vi "Mojo Engine.vi"(0 "Mojo Notifier":string, 11 "COM Port":string[](array[string])) -> ()   [LabVIEW 2020]
uses:
  FPGA Controls/FPGA Cluster.ctl
  FPGA Controls/FPGA Laser Mode.ctl
  FPGA Controls/FPGA Sequence Mode.ctl
  FPGA Controls/FPGA Notifier Element.ctl
  FPGA Controls/FPGA Action.ctl
panel:
  in  "488":T1 {"Duration digital" max=65535 step=1; "Duration slide" max=65535 step=1 scale=0.0..65535.0 scale format="%d us"; "Laser Mode" items=["Off", "On", "Rising", "Falling", "Camera"]}
  in  "405":T1 {"Duration digital" max=65535 step=1; "Duration slide" max=65535 step=1 scale=0.0..65535.0 scale format="%d us"; "Laser Mode" items=["Off", "On", "Rising", "Falling", "Camera"]}
  out "Startup Error":errorcluster
  in  "Quit":bool
  out "Version":u32
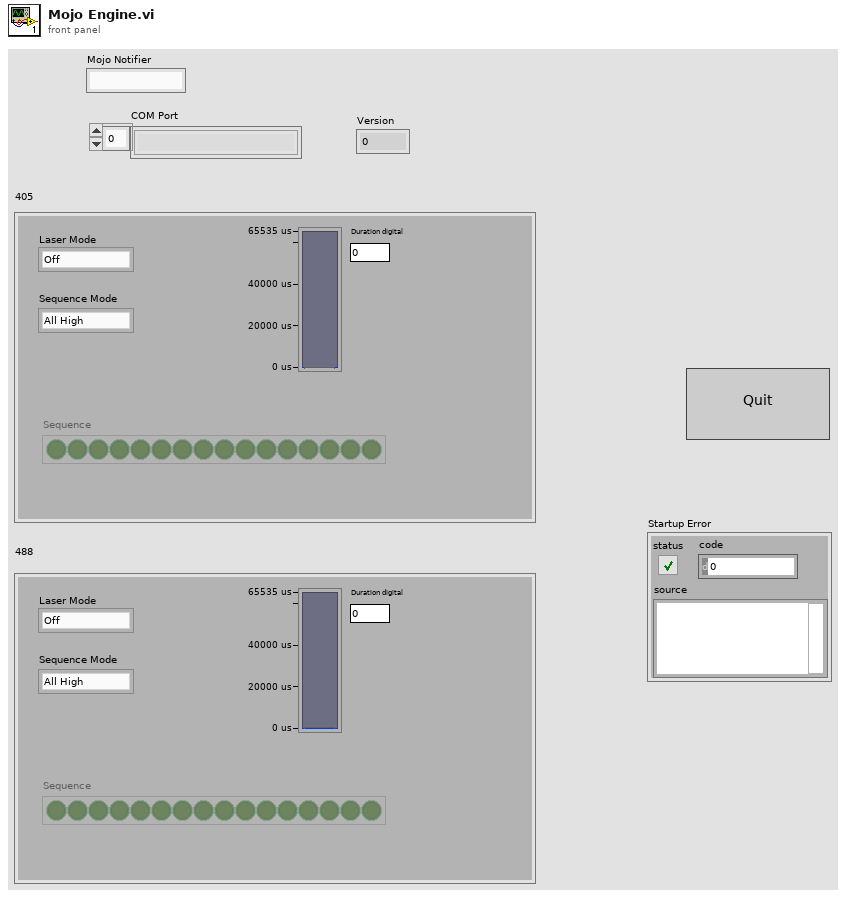
[diagram p1: front panel]
types:
  T1 = typedef "FPGA Cluster.ctl" = cluster{"Laser Mode":T2, "Sequence Mode":T3, "Duration slide":u32, "Duration digital":u32, "Sequence":bool[]}
  T2 = typedef "FPGA Laser Mode.ctl" = u16
  T3 = typedef "FPGA Sequence Mode.ctl" = enum16{"All High", "All Low", "Alternate 1010", "Alternate 0101", "Custom"}
  T4 = enum8{"Enabled", "Disabled", "Disabled and Grayed Out"}
  T5 = typedef "FPGA Notifier Element.ctl" = cluster{"Sequence":bool[], "Laser Mode":T2, "Duration":u32, "Laser Channel":u16, "Write Confirm ":bool, "Received?":bool, "FPGA Action":T6}
  T6 = typedef "FPGA Action.ctl" = enum16{"Set Laser Mode", "Set Sequence", "Set Duration", "Write Check", "Idle", "Quit"}
  T7 = enum16{"All High", "All Low", "Alternate 1010", "Alternate 0101", "Custom"}
  T8 = cluster{"Laser Mode":bool, "Sequence Mode":bool, "Duration slide":bool, "Duration digital":bool, "Sequence":bool[]}
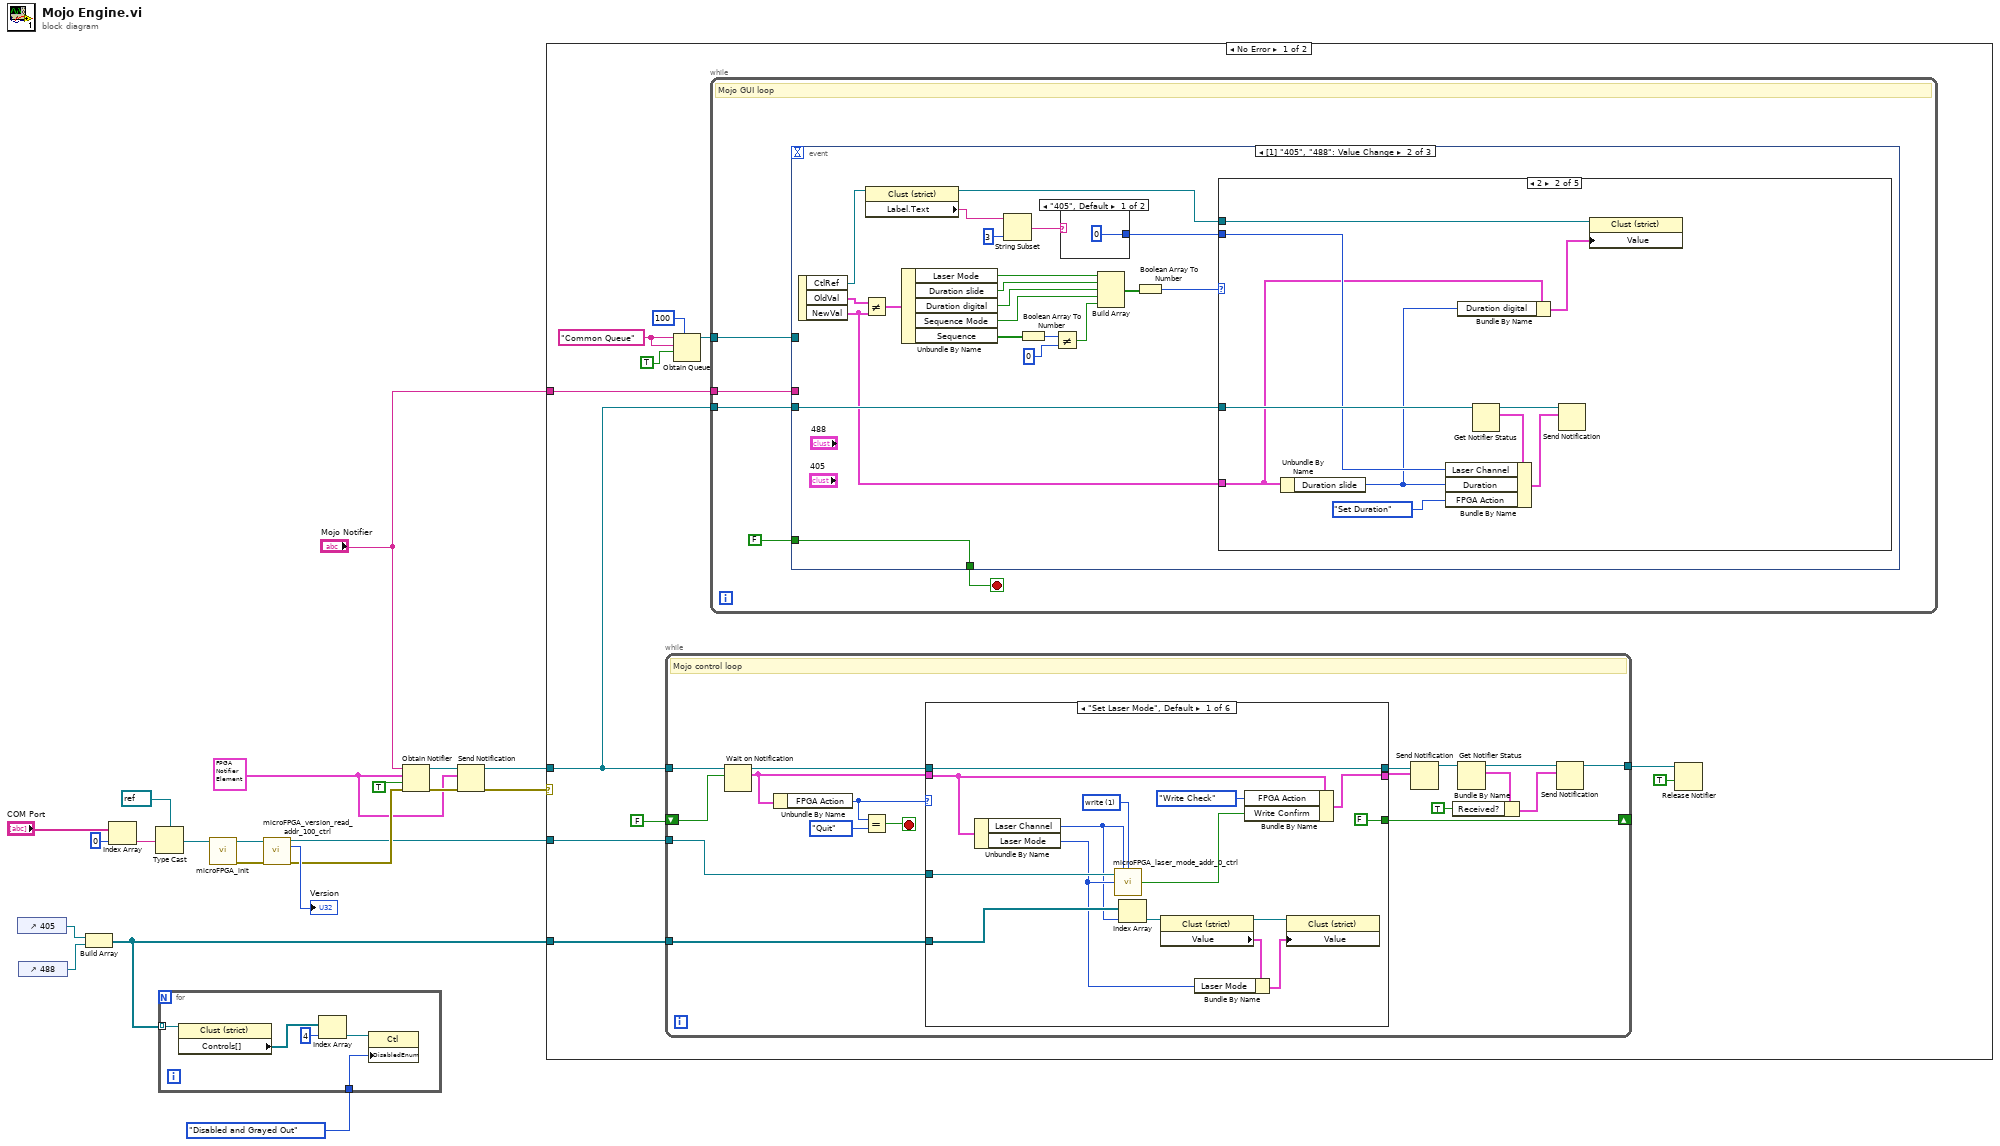
[diagram p0: block diagram]
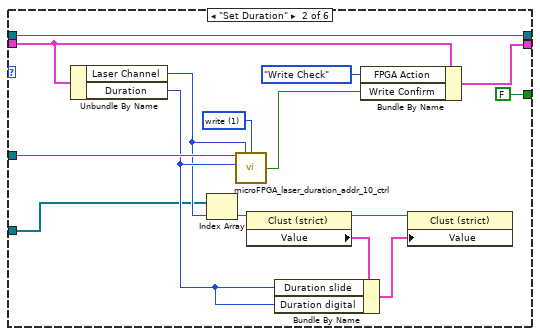
[diagram p2: hidden frame]
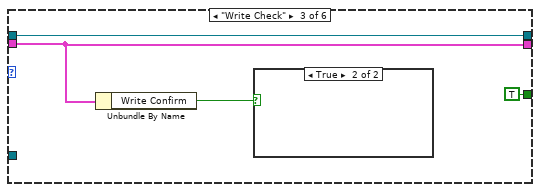
[diagram p3: hidden frame]
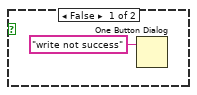
[diagram p4: hidden frame]
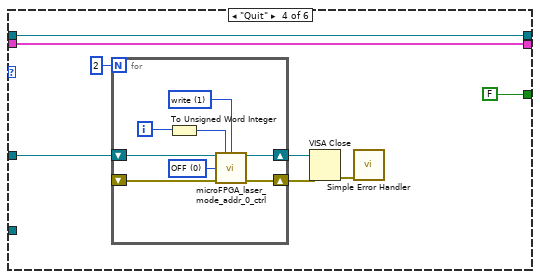
[diagram p5: hidden frame]
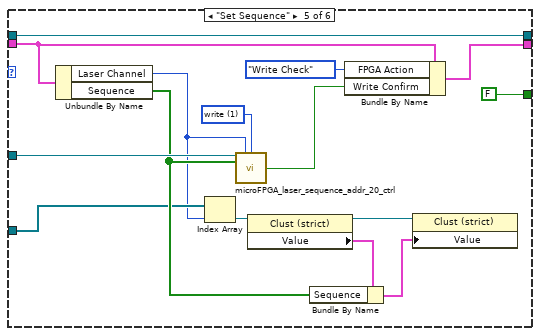
[diagram p6: hidden frame]
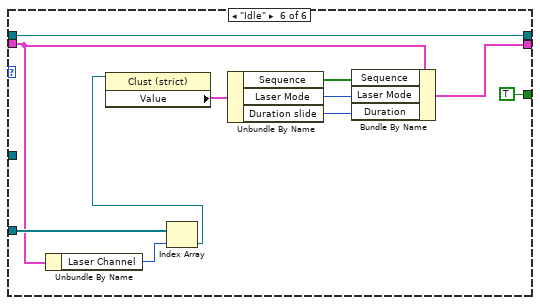
[diagram p7: hidden frame]
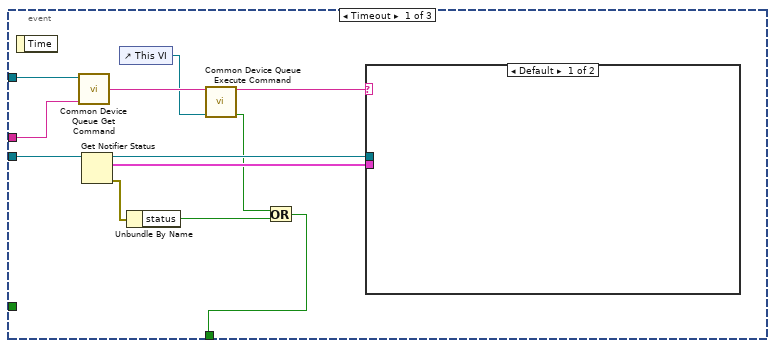
[diagram p8: hidden frame]
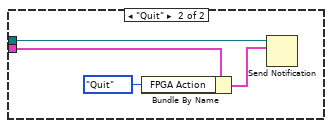
[diagram p9: hidden frame]
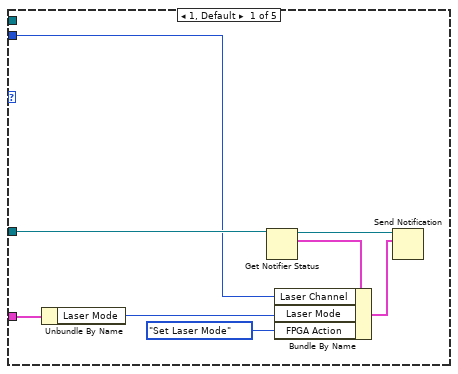
[diagram p10: hidden frame]
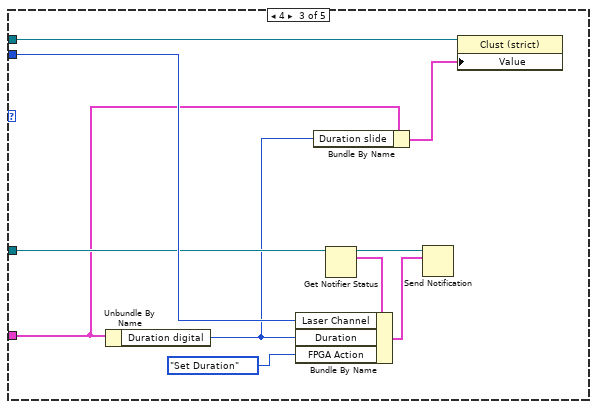
[diagram p11: hidden frame]
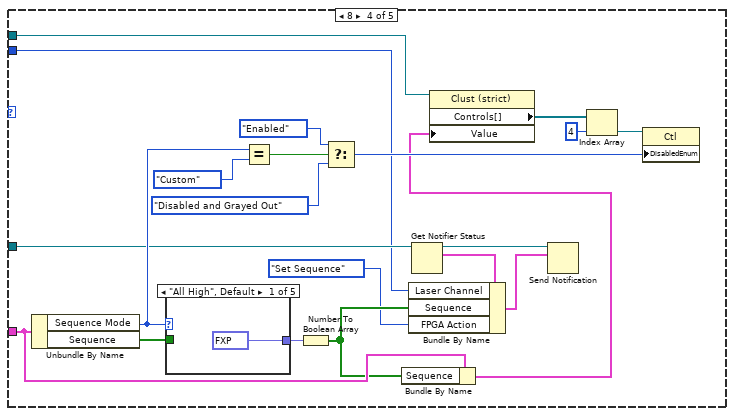
[diagram p12: hidden frame]
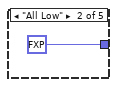
[diagram p13: hidden frame]
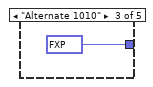
[diagram p14: hidden frame]
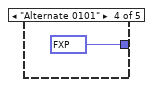
[diagram p15: hidden frame]
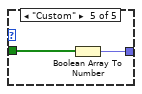
[diagram p16: hidden frame]
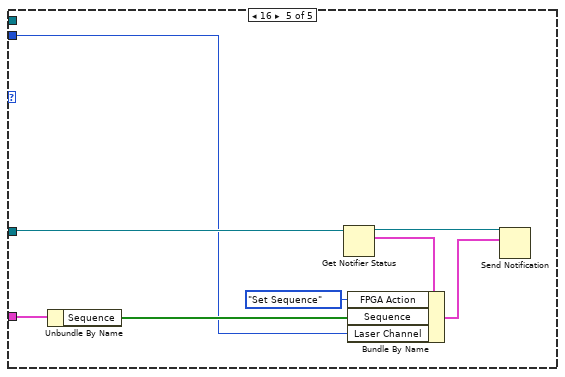
[diagram p17: hidden frame]
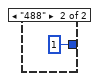
[diagram p18: hidden frame]
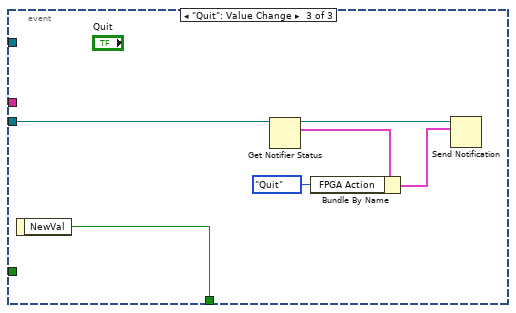
[diagram p19: hidden frame]
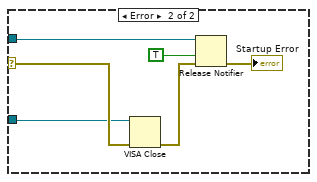
[diagram p20: hidden frame]
diagram:
  w5 = T5 {"Sequence"=[FALSE, FALSE, FALSE, FALSE, FALSE, FALSE, FALSE, FALSE, FALSE, FALSE, FALSE, FALSE, FALSE, FALSE, FALSE, FALSE], "Laser Mode"=0, "Duration"=0, "Laser Channel"=0, "Write Confirm "=FALSE, "Received?"=FALSE, "FPGA Action"=enum."Idle"} ("Mojo Notifier Element")
  n1 = control-ref of="405"() -> (w4:refnum<vi>)
  n2 = control-ref of="488"() -> (w3:refnum<vi>)
  n3 = Build Array(w4, w3) -> (w1:refnum<vi>[])
  n4 = Index Array(array="COM Port", index=0) -> (element=w19:string)
  n5 = Type Cast(type=refnum<visa-resource-name> refnum ("VISA resource name"), x=w19) -> (*(type *) &x=w17:refnum<visa-resource-name>)
  n6 = for {
    tunnel: w1 -> [w24] mode=indexing
    tunnel: T4."Disabled and Grayed Out" ("Disabled") -> [w22]
    n7 = property class="Clust (strict)"(reference=w24) -> ("Controls[]"=w23:refnum<vi>[])  [unwired: 1 in, 2 out]
    n8 = Index Array(array=w23, index=4) -> (element=w25:refnum<vi>)
    n9 = property class="Ctl"(reference=w25, "DisabledEnum"=w22) -> ()  [unwired: 1 in, 2 out]
  }
  n10 = call "microFPGA_init.vi"("VISA resource name"=w17) -> ("error out"=w15:errorcluster, "VISA resource name out"=w16:refnum<visa-resource-name>)  [unwired: 9 in]
  n11 = call "microFPGA_version_read_addr_100_ctrl.vi"("VISA resource name"=w16, "error in (no error)"=w15) -> ("VISA resource name out"=w7:refnum<visa-resource-name>, "Version"=→"Version":u32, "error out"=w13:errorcluster)  [unwired: 11 in]
  n12 = Obtain Notifier(name (unnamed)="Mojo Notifier", notification data type=w5, create if not found? (T)=TRUE, error in (no error)=w13) -> (notifier out=w11:refnum<notifier>, error out=w10:errorcluster)  [unwired: 1 out]
  n13 = Send Notification(notification=w5, notifier=w11, error in (no error)=w10) -> (notifier out=w8:refnum<notifier>, error out=w9:errorcluster)
  n14 = case shown="No Error" w9 {
    selector: w9 -> [_ w247]
    tunnel: w8 -> [w37 w248]
    tunnel: w7 -> [w36 w246]
    tunnel: "Mojo Notifier" -> [w29 _]
    tunnel: w1 -> [w27 _]
    frame No Error {
      w33 = "Common Queue" ("Unique Notifier Name")
      n15 = while {
        tunnel: w37 -> [w55]
        tunnel: w36 -> [w50]
        tunnel: [w42] -> w35
        shift-right: [w47] -> _
        shift-left: FALSE -> [w46]
        tunnel: w27 -> [w38]
        stop <- w51 stop-if-true
        # "Mojo control loop"
        n16 = Wait on Notification(notifier=w55, ignore previous (F)=w46) -> (notifier out=w53:refnum<notifier>, notification=w52:T5)  [unwired: 2 in, 2 out]
        n17 = Unbundle By Name(w52) -> ("FPGA Action"=w54:T6)
        n18 = Equal?(x=w54, y=FPGA_Action."Quit") -> (x = y?=w51:bool)
        n19 = case shown="\"Set Laser Mode\", Default" w54 {
          tunnel: w53 -> [w67 w84 w87 w97 w120 w132]
          tunnel: w52 -> [w68 w83 w88 w96 w119 w126]
          tunnel: w50 -> [w70 w81 _ w94 w117 _]
          tunnel: [w67 w84 w87 w97 w120 w132] -> w49
          tunnel: [w65 w85 w88 w96 w121 w122] -> w48
          tunnel: [FALSE FALSE TRUE FALSE FALSE TRUE] -> w47
          tunnel: w38 -> [w62 w74 _ _ w111 w130]
          frame "Set Laser Mode", Default {
            w69 = u16 1 items=["read", "write"] ("write or read")
            n20 = Unbundle By Name(w68) -> ("Laser Channel"=w60:u16, "Laser Mode"=w61:T2)
            n21 = call "microFPGA_laser_mode_addr_0_ctrl.vi"("VISA resource name"=w70, "laser channel"=w60, "write or read"=w69, "laser mode write"=w61) -> ("value write confirm"=w66:bool)  [unwired: 7 in, 4 out]
            n22 = Index Array(array=w62, index=w60) -> (element=w58:refnum<vi>)
            n23 = property class="Clust (strict)"(reference=w58) -> (reference out=w56:refnum<vi>, "Value"=w57:T1)  [unwired: 1 in, 1 out]
            n24 = Bundle By Name(cluster=w57, "Laser Mode"=w61) -> (w59:T1)
            n25 = Bundle By Name(cluster=w68, "FPGA Action"=FPGA_Action."Write Check", "Write Confirm"=w66) -> (w65:T5)
            n26 = property class="Clust (strict)"(reference=w56, "Value"=w59) -> ()  [unwired: 1 in, 2 out]
          }
          frame "Set Duration" {
            w82 = u16 1 items=["read", "write"] ("write or read")
            n27 = Unbundle By Name(w83) -> ("Laser Channel"=w75:u16, "Duration"=w76:u32)
            n28 = Index Array(array=w74, index=w75) -> (element=w73:refnum<vi>)
            n29 = call "microFPGA_laser_duration_addr_10_ctrl.vi"("VISA resource name"=w81, "laser channel"=w75, "write or read"=w82, "duration write"=w76) -> ("value write confirm"=w80:bool)  [unwired: 7 in, 4 out]
            n30 = property class="Clust (strict)"(reference=w73) -> (reference out=w71:refnum<vi>, "Value"=w72:T1)  [unwired: 1 in, 1 out]
            n31 = Bundle By Name(cluster=w72, "Duration slide"=w76, "Duration digital"=w76) -> (w77:T1)
            n32 = Bundle By Name(cluster=w83, "FPGA Action"=FPGA_Action."Write Check", "Write Confirm"=w80) -> (w85:T5)
            n33 = property class="Clust (strict)"(reference=w71, "Value"=w77) -> ()  [unwired: 1 in, 2 out]
          }
          frame "Write Check" {
            n34 = Unbundle By Name(w88) -> ("Write Confirm"=w89:bool)
            n35 = case shown="True" w89 {
              frame False {
                n36 = One Button Dialog(message="write not success") -> ()  [unwired: 1 in, 1 out]
              }
              frame True {
              }
            }
          }
          frame "Quit" {
            n37 = for {
              N: 2 -> [_]
              shift-right: [w105] -> w93
              shift-left: w94 -> [w106]
              shift-right: [w104] -> w92
              shift-left: _ -> [w102]
              i -> [w101]
              w99 = u16 0 items=["OFF", "ON", "RISING", "FALLING", "CAMERA"] ("laser mode write")
              w103 = u16 1 items=["read", "write"] ("write or read")
              n38 = To Unsigned Word Integer(number=w101) -> (unsigned 16bit integer=w100:u16)
              n39 = call "microFPGA_laser_mode_addr_0_ctrl.vi"("VISA resource name"=w106, "laser channel"=w100, "write or read"=w103, "laser mode write"=w99, "error in (no error)"=w102) -> ("VISA resource name out"=w105:refnum<visa-resource-name>, "error out"=w104:errorcluster)  [unwired: 6 in, 3 out]
            }
            n40 = VISA Close(VISA resource name=w93, error in (no error)=w92) -> (error out=w98:errorcluster)
            n41 = call <vilib>:"Simple Error Handler.vi"("error in (no error)"=w98) -> ()  [unwired: 4 in, 5 out]
          }
          frame "Set Sequence" {
            w118 = u16 1 items=["read", "write"] ("write or read")
            n42 = Unbundle By Name(w119) -> ("Laser Channel"=w110:u16, "Sequence"=w112:bool[])
            n43 = Index Array(array=w111, index=w110) -> (element=w109:refnum<vi>)
            n44 = call "microFPGA_laser_sequence_addr_20_ctrl.vi"("VISA resource name"=w117, "laser channel"=w110, "write or read"=w118, "sequence write"=w112) -> ("value write confirm"=w116:bool)  [unwired: 7 in, 4 out]
            n45 = property class="Clust (strict)"(reference=w109) -> (reference out=w107:refnum<vi>, "Value"=w108:T1)  [unwired: 1 in, 1 out]
            n46 = Bundle By Name(cluster=w108, "Sequence"=w112) -> (w113:T1)
            n47 = Bundle By Name(cluster=w119, "FPGA Action"=FPGA_Action."Write Check", "Write Confirm"=w116) -> (w121:T5)
            n48 = property class="Clust (strict)"(reference=w107, "Value"=w113) -> ()  [unwired: 1 in, 2 out]
          }
          frame "Idle" {
            n49 = Unbundle By Name(w126) -> ("Laser Channel"=w129:u16)
            n50 = Index Array(array=w130, index=w129) -> (element=w127:refnum<vi>)
            n51 = property class="Clust (strict)"(reference=w127) -> ("Value"=w128:T1)  [unwired: 1 in, 2 out]
            n52 = Unbundle By Name(w128) -> ("Sequence"=w125:bool[], "Laser Mode"=w124:T2, "Duration slide"=w123:u32)
            n53 = Bundle By Name(cluster=w126, "Sequence"=w125, "Laser Mode"=w124, "Duration"=w123) -> (w122:T5)
          }
        }
        n54 = Send Notification(notification=w48, notifier=w49) -> (notifier out=w45:refnum<notifier>)  [unwired: 1 in, 1 out]
        n55 = Get Notifier Status(notifier=w45) -> (notifier out=w43:refnum<notifier>, current notification=w44:T5)  [unwired: 1 in, 3 out]
        n56 = Bundle By Name(cluster=w44, "Received?"=TRUE) -> (w41:T5)
        n57 = Send Notification(notification=w41, notifier=w43) -> (notifier out=w42:refnum<notifier>)  [unwired: 1 in, 1 out]
      }
      n58 = Obtain Queue(max queue size (-1, unlimited)=100, name (unnamed)=w33, element data type=w33, create if not found? (T)=TRUE) -> (queue out=w30:refnum<queue>)  [unwired: 1 in, 2 out]
      n59 = while {
        tunnel: w37 -> [w136]
        tunnel: w30 -> [w134]
        tunnel: w29 -> [w133]
        stop <- w135 stop-if-true
        # "Mojo GUI loop"
        n60 = event shown="[1] \"405\", \"488\": Value Change" {
          selector: _ -> [_ _ _]
          dyn-events: _ -> [_ _ _]
          timeout: _ -> [_ _ _]
          tunnel: FALSE -> [_ w154 _]
          tunnel: w136 -> [w144 w158 w244]
          tunnel: [w138 w154 w245] -> w135
          tunnel: w134 -> [w149 _ _]
          tunnel: w133 -> [w148 _ _]
          event Timeout {
            n61 = event-data() -> ()  [unwired: 1 in, 1 out]
            n62 = call "Common Device Queue Get Command.vi"("Common Queue"=w149, "Notifier Name"=w148) -> ("Command"=w147:string)  [unwired: 12 in, 1 out]
            n63 = Get Notifier Status(notifier=w144) -> (notifier out=w143:refnum<notifier>, current notification=w142:T5, error out=w141:errorcluster)  [unwired: 1 in, 2 out]
            n64 = control-ref of="This VI"() -> (w146:refnum<vi>)
            n65 = Unbundle By Name(w141) -> ("status"=w139:bool)
            n66 = call "Common Device Queue Execute Command.vi"("Common Command"=w147, "VI Refnum"=w146) -> ("Common Command"=w145:string, "Quit?"=w140:bool)  [unwired: 12 in]
            n67 = Or(x=w140, y=w139) -> (x .or. y?=w138:bool)
            n68 = case shown="Default" w145 {
              tunnel: w143 -> [_ w153]
              tunnel: w142 -> [_ w152]
              frame Default {
              }
              frame "Quit" {
                n69 = Bundle By Name(cluster=w152, "FPGA Action"=FPGA_Action."Quit") -> (w151:T5)
                n70 = Send Notification(notification=w151, notifier=w153) -> ()  [unwired: 1 in, 2 out]
              }
            }
          }
          event Value Change {
            n71 = event-data() -> ("CtlRef"=w163:refnum<vi>, "OldVal"=w164:T1, "NewVal"=w156:T1)  [unwired: 1 in]
            n72 = Not Equal?(x=w164, y=w156) -> (x != y?=w165:T8)
            n73 = property class="Clust (strict)"(reference=w163) -> (reference out=w155:refnum<vi>, "Label.Text"=w160:string)  [unwired: 1 in, 1 out]
            n74 = Unbundle By Name(w165) -> ("Laser Mode"=w169:bool, "Duration slide"=w170:bool, "Duration digital"=w171:bool, "Sequence Mode"=w172:bool, "Sequence"=w166:bool[])
            n75 = String Subset(string=w160, length (rest)=3 ("length (rest)")) -> (substring=w161:string)  [unwired: 1 in]
            n76 = Boolean Array To Number(Boolean array=w166) -> (number=w167:u32)
            n77 = Not Equal?(x=w167, y=u32 0) -> (x != y?=w173:bool)
            n78 = case shown="\"405\", Default" w161 {
              tunnel: [u16 0 ("Laser Channel") u16 1 ("Laser Channel")] -> w157
              frame "405", Default {
              }
              frame "488" {
              }
            }
            n79 = Build Array(w169, w170, w171, w172, w173) -> (w174:bool[])
            n80 = Boolean Array To Number(Boolean array=w174) -> (number=w159:u32)
            n81 = case shown="2" w159 {
              tunnel: w158 -> [w178 w189 w195 w205 w233]
              tunnel: w157 -> [w177 w187 w196 w203 w230]
              tunnel: w156 -> [w176 w186 w194 w209 w232]
              tunnel: w155 -> [_ w185 w197 w210 _]
              frame 1, Default {
                n82 = Unbundle By Name(w176) -> ("Laser Mode"=w175:T2)
                n83 = Get Notifier Status(notifier=w178) -> (notifier out=w181:refnum<notifier>, current notification=w180:T5)  [unwired: 1 in, 3 out]
                n84 = Bundle By Name(cluster=w180, "Laser Channel"=w177, "Laser Mode"=w175, "FPGA Action"=FPGA_Action."Set Laser Mode") -> (w182:T5)
                n85 = Send Notification(notification=w182, notifier=w181) -> ()  [unwired: 1 in, 2 out]
              }
              frame 2 {
                n86 = Unbundle By Name(w186) -> ("Duration slide"=w183:u32)
                n87 = Bundle By Name(cluster=w186, "Duration digital"=w183) -> (w184:T1)
                n88 = Get Notifier Status(notifier=w189) -> (notifier out=w192:refnum<notifier>, current notification=w190:T5)  [unwired: 1 in, 3 out]
                n89 = Bundle By Name(cluster=w190, "Laser Channel"=w187, "Duration"=w183, "FPGA Action"=FPGA_Action."Set Duration") -> (w191:T5)
                n90 = Send Notification(notification=w191, notifier=w192) -> ()  [unwired: 1 in, 2 out]
                n91 = property class="Clust (strict)"(reference=w185, "Value"=w184) -> ()  [unwired: 1 in, 2 out]
              }
              frame 4 {
                n92 = Unbundle By Name(w194) -> ("Duration digital"=w193:u32)
                n93 = Bundle By Name(cluster=w194, "Duration slide"=w193) -> (w198:T1)
                n94 = Get Notifier Status(notifier=w195) -> (notifier out=w202:refnum<notifier>, current notification=w200:T5)  [unwired: 1 in, 3 out]
                n95 = Bundle By Name(cluster=w200, "Laser Channel"=w196, "Duration"=w193, "FPGA Action"=FPGA_Action."Set Duration") -> (w201:T5)
                n96 = Send Notification(notification=w201, notifier=w202) -> ()  [unwired: 1 in, 2 out]
                n97 = property class="Clust (strict)"(reference=w197, "Value"=w198) -> ()  [unwired: 1 in, 2 out]
              }
              frame 8 {
                n98 = Unbundle By Name(w209) -> ("Sequence Mode"=w206:T3, "Sequence"=w215:bool[])
                n99 = case shown="\"All High\", Default" w206 {
                  tunnel: [fxp<+,16,16> 65535.0 ("number") fxp<+,16,16> 0.0 ("number") fxp<+,16,16> 43690.0 ("number") fxp<+,16,16> 21845.0 ("number") w229] -> w216
                  tunnel: w215 -> [_ _ _ _ w228]
                  frame "All High", Default {
                  }
                  frame "All Low" {
                  }
                  frame "Alternate 1010" {
                  }
                  frame "Alternate 0101" {
                  }
                  frame "Custom" {
                    n100 = Boolean Array To Number(Boolean array=w228) -> (number=w229:fxp<+,16,16>)
                  }
                }
                n101 = Equal?(x=w206, y=T7."Custom") -> (x = y?=w222:bool)
                n102 = Number To Boolean Array(number=w216) -> (Boolean array=w208:bool[])
                n103 = Select(t=T4."Enabled" ("Disabled"), s=w222, f=T4."Disabled and Grayed Out") -> (s? t:f=w211:T4)
                n104 = Bundle By Name(cluster=w209, "Sequence"=w208) -> (w207:T1)
                n105 = Get Notifier Status(notifier=w205) -> (notifier out=w219:refnum<notifier>, current notification=w218:T5)  [unwired: 1 in, 3 out]
                n106 = Bundle By Name(cluster=w218, "Laser Channel"=w203, "Sequence"=w208, "FPGA Action"=FPGA_Action."Set Sequence") -> (w217:T5)
                n107 = property class="Clust (strict)"(reference=w210, "Value"=w207) -> ("Controls[]"=w214:refnum<vi>[])  [unwired: 1 in, 2 out]
                n108 = Send Notification(notification=w217, notifier=w219) -> ()  [unwired: 1 in, 2 out]
                n109 = Index Array(array=w214, index=4) -> (element=w212:refnum<vi>)
                n110 = property class="Ctl"(reference=w212, "DisabledEnum"=w211) -> ()  [unwired: 1 in, 2 out]
              }
              frame 16 {
                n111 = Unbundle By Name(w232) -> ("Sequence"=w231:bool[])
                n112 = Get Notifier Status(notifier=w233) -> (notifier out=w236:refnum<notifier>, current notification=w237:T5)  [unwired: 1 in, 3 out]
                n113 = Bundle By Name(cluster=w237, "FPGA Action"=FPGA_Action."Set Sequence", "Sequence"=w231, "Laser Channel"=w230) -> (w235:T5)
                n114 = Send Notification(notification=w235, notifier=w236) -> ()  [unwired: 1 in, 2 out]
              }
            }
          }
          event "Quit": Value Change {
            n115 = event-data() -> ("NewVal"=w245:bool)  [unwired: 1 in]
            n116 = Get Notifier Status(notifier=w244) -> (notifier out=w242:refnum<notifier>, current notification=w243:T5)  [unwired: 1 in, 3 out]
            n117 = Bundle By Name(cluster=w243, "FPGA Action"=FPGA_Action."Quit") -> (w241:T5)
            n118 = Send Notification(notification=w241, notifier=w242) -> ()  [unwired: 1 in, 2 out]
          }
        }
      }
      n119 = Release Notifier(notifier=w35, force destroy? (F)=TRUE) -> ()  [unwired: 1 in, 3 out]
    }
    frame Error {
      n120 = VISA Close(VISA resource name=w246, error in (no error)=w247) -> (error out=w250:errorcluster)
      n121 = Release Notifier(notifier=w248, force destroy? (F)=TRUE, error in (no error)=w250) -> (error out=→"Startup Error":errorcluster)  [unwired: 2 out]
    }
  }
